vi "LS372_serial_write.vi"(8 "error in (no error)":errorcluster {"code" format="%.0x"}, 10 "Write Buffer (\"\")":string, 11 "VISA resource name":refnum<visa-resource-name>) -> (0 "error out":errorcluster {"code" format="%.0x"}, 2 "Return Count":u32, 3 "VISA resource name out":refnum<visa-resource-name>)   [LabVIEW 2018]
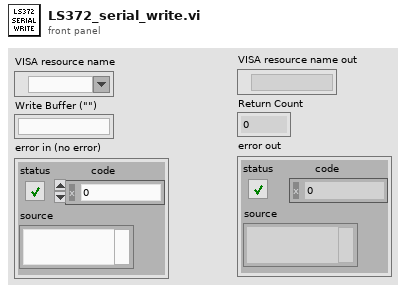
[diagram p1: front panel]
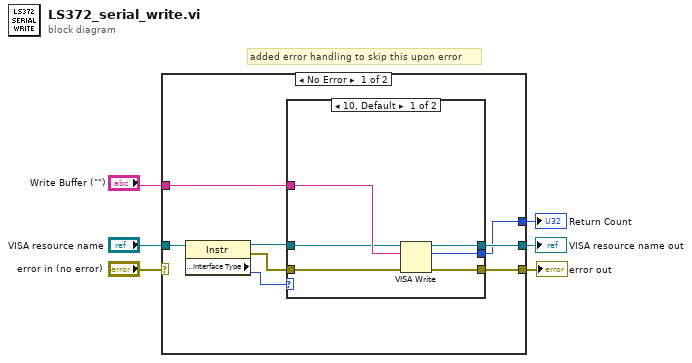
[diagram p0: block diagram]
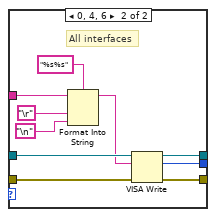
[diagram p2: hidden frame]
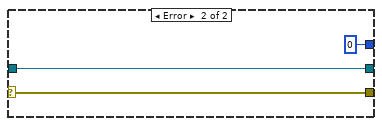
[diagram p3: hidden frame]
diagram:
  # "added error handling to skip this upon error"
  n1 = case shown="No Error" "error in (no error)" {
    selector: "error in (no error)" -> [_ w32]
    tunnel: [w14 w32] -> w6
    tunnel: [w13 w33] -> w5
    tunnel: [w12 u32 0 ("return count")] -> w1
    tunnel: "Write Buffer (\"\")" -> [w11 _]
    tunnel: "VISA resource name" -> [w10 w33]
    frame No Error {
      n2 = property class="Instr"(reference=w10) -> (reference out=w8:refnum<visa-resource-name>, error out=w9:errorcluster, "Interface Information:Interface Type"=w7:u16)  [unwired: 1 in]
      n3 = case shown="10, Default" w7 {
        tunnel: [w17 w30] -> w14
        tunnel: [w16 w29] -> w13
        tunnel: [w15 w28] -> w12
        tunnel: w8 -> [w19 w27]
        tunnel: w9 -> [w18 w26]
        tunnel: w11 -> [w20 w25]
        frame 10, Default {
          n4 = VISA Write(VISA resource name=w19, write buffer=w20, error in (no error)=w18) -> (VISA resource name out=w16:refnum<visa-resource-name>, return count=w15:u32, error out=w17:errorcluster)
        }
        frame 0, 4, 6 {
          # "All interfaces"
          n5 = Format Into String(format string="%s%s", initial string=w25, "\r", "\n") -> (resulting string=w21:string)  [unwired: 1 in, 1 out]
          n6 = VISA Write(VISA resource name=w27, write buffer=w21, error in (no error)=w26) -> (VISA resource name out=w29:refnum<visa-resource-name>, return count=w28:u32, error out=w30:errorcluster)
        }
      }
    }
    frame Error {
    }
  }
  "VISA resource name out" <- w5
  "error out" <- w6
  "Return Count" <- w1
